vi "Build Results.vi"(6 "Score":dbl, 8 "Center":T1, 9 "Distance":dbl, 10 "Bounding Box":T5 {"Bottom" format="%#_3g"; "Right" format="%#_3g"; "Top" format="%#_3g"; "Left" format="%#_3g"}, 11 "Image":T2) -> (1 "Results Out":T3 {"Score" format="%#_3g"; "Pixels"."Box"."Bottom" format="%#_3g"; "Pixels"."Box"."Right" format="%#_3g"; "Pixels"."Box"."Top" format="%#_3g"; "Pixels"."Box"."Left" format="%#_3g"; "Normalized"."Box"."Bottom" format="%#_3g"; "Normalized"."Box"."Right" format="%#_3g"; "Normalized"."Box"."Top" format="%#_3g"; "Normalized"."Box"."Left" format="%#_3g"; "Distance (ft)" format="%#_3g"}, 3 "Image Out":T2)   [LabVIEW 2017, in "VisionSystem.lvlib"]
doc: "Normalize the rectangle and center so that they range from -1 to 1, left to right and bottom to top. This helps with producing joystick coordinates for driving the robot and makes the code better at handling resolution changes of the camera."
uses:
  VisionSystem.lvlib
  <vilib>/vision/Image Controls.llb/IMAQ Image.ctl
  Cluster_UI DBL Box.ctl
  Cluster_Results.ctl
  Cluster_Targeting Data.ctl
  Cluster_SGL Point.ctl
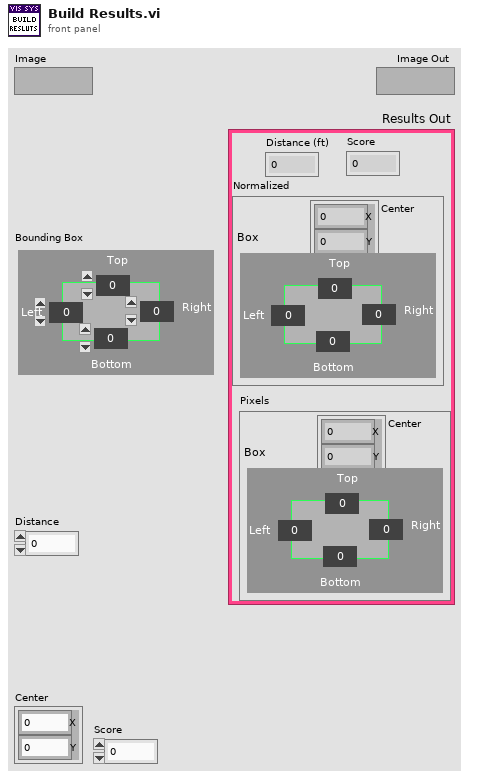
[diagram p1: front panel]
types:
  T1 = typedef "VisionSystem.lvlib/Cluster_SGL Point.ctl" = cluster{"X":sgl, "Y":sgl}
  T2 = typedef "IMAQ Image.ctl" = refnum<image>
  T3 = typedef "VisionSystem.lvlib/Cluster_Results.ctl" = cluster{"Distance (ft)":dbl, "Score":dbl, "Normalized":T4, "Pixels":T4}
  T4 = typedef "VisionSystem.lvlib/Cluster_Targeting Data.ctl" = cluster{"Center":T1, "Box":T5}
  T5 = typedef "VisionSystem.lvlib/Cluster_UI DBL Box.ctl" = cluster{"Left":dbl, "Top":dbl, "Right":dbl, "Bottom":dbl}
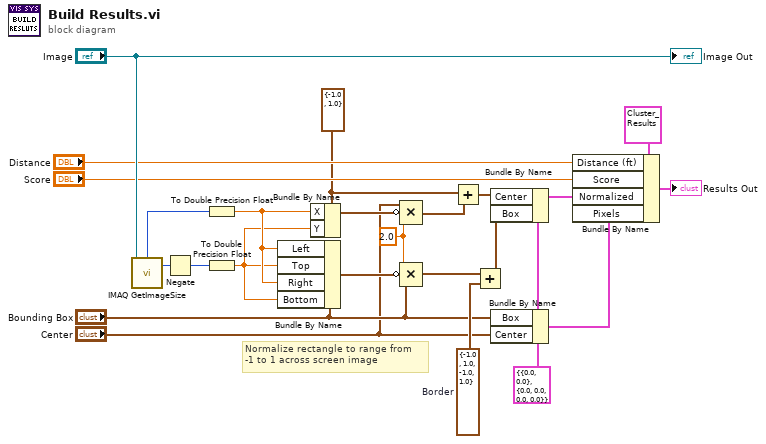
[diagram p0: block diagram]
diagram:
  w6 = T4 {"Center"={"X"=0.0, "Y"=0.0}, "Box"={"Left"=0.0, "Top"=0.0, "Right"=0.0, "Bottom"=0.0}} ("Vision Targeting Data")
  w3 = T1 {"X"=-1.0, "Y"=1.0} ("y")
  w12 = 2.0
  w23 = T5 {"Left"=-1.0, "Top"=1.0, "Right"=-1.0, "Bottom"=1.0}  # Border
  # "Normalize rectangle to range from\n-1 to 1 across screen image"
  n1 = call "IMAQ GetImageSize"("Image"="Image") -> ("Y Resolution"=w24:i32, "X Resolution"=w15:i32)  [unwired: 3 in, 1 out]
  n2 = Negate(x=w24) -> (-x=w14:i32)
  n3 = To Double Precision Float(number=w15) -> (double precision float=w5:dbl)
  n4 = To Double Precision Float(number=w14) -> (double precision float=w4:dbl)
  n5 = Bundle By Name(cluster="Bounding Box", "Left"=w5, "Top"=w4, "Right"=w5, "Bottom"=w4) -> (w22:T5)
  n6 = Bundle By Name(cluster=w3, "X"=w5, "Y"=w4) -> (w13:T1)
  n7 = Compound Arithmetic op=MULTIPLY("Center", invert w13, w12) -> (w11:cluster{"X":dbl, "Y":dbl})
  n8 = Compound Arithmetic op=MULTIPLY(w12, invert w22, "Bounding Box") -> (w21:T5)
  n9 = Add(x=w3, y=w11) -> (x+y=w10:cluster{"X":dbl, "Y":dbl})
  n10 = Add(x=w21, y=w23) -> (x+y=w20:T5)
  n11 = Bundle By Name(cluster=w6, "Center"=w10, "Box"=w20) -> (w18:T4)
  n12 = Bundle By Name(cluster=w6, "Box"="Bounding Box", "Center"="Center") -> (w16:T4)
  n13 = Bundle By Name(cluster=T3 {"Distance (ft)"=0.0, "Score"=0.0, "Normalized"={"Center"={"X"=0.0, "Y"=0.0}, "Box"={"Left"=0.0, "Top"=0.0, "Right"=0.0, "Bottom"=0.0}}, "Pixels"={"Center"={"X"=0.0, "Y"=0.0}, "Box"={"Left"=0.0, "Top"=0.0, "Right"=0.0, "Bottom"=0.0}}} ("Results Out"), "Distance (ft)"="Distance", "Score"="Score", "Normalized"=w18, "Pixels"=w16) -> (→"Results Out":T3)
  "Image Out" <- "Image"
